vi "Configure Outputs.vi"(0 "VISA resource name":refnum<visa-resource-name>, 1 "Analog Bandwidth (0: bw200kHz)":i32(ring) items=["bw200kHz", "bw50kHz", "bw25kHz"], 2 "Sample Rate (24000 Hz)":dbl=24000.0, 5 "Domain (0: odAnalog)":i32(ring) items=["odAnalog", "odDigital", "odExternal"], 7 "Channels (1)":i32=1, 9 "Connector Type (0: cXLR)":i32(ring) items=["cXLR", "cBNC", "cOptical"], 11 "error in (no error)":errorcluster, 12 "Enable Digital Dual Connector (T: Enable)":bool=TRUE) -> (4 "VISA resource name out":refnum<visa-resource-name>, 15 "error out":errorcluster)   [LabVIEW 2014, in "Stanford Research SR1.lvlib"]
doc: "Configures the attributes for the Quick Measurement Outputs."
uses:
  Stanford Research SR1.lvlib
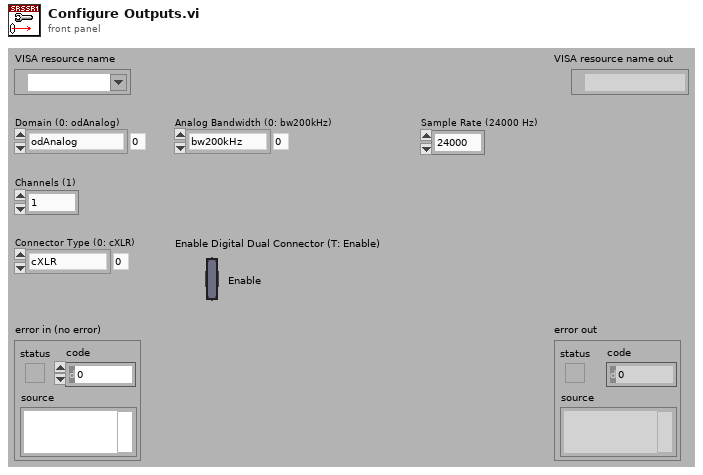
[diagram p1: front panel]
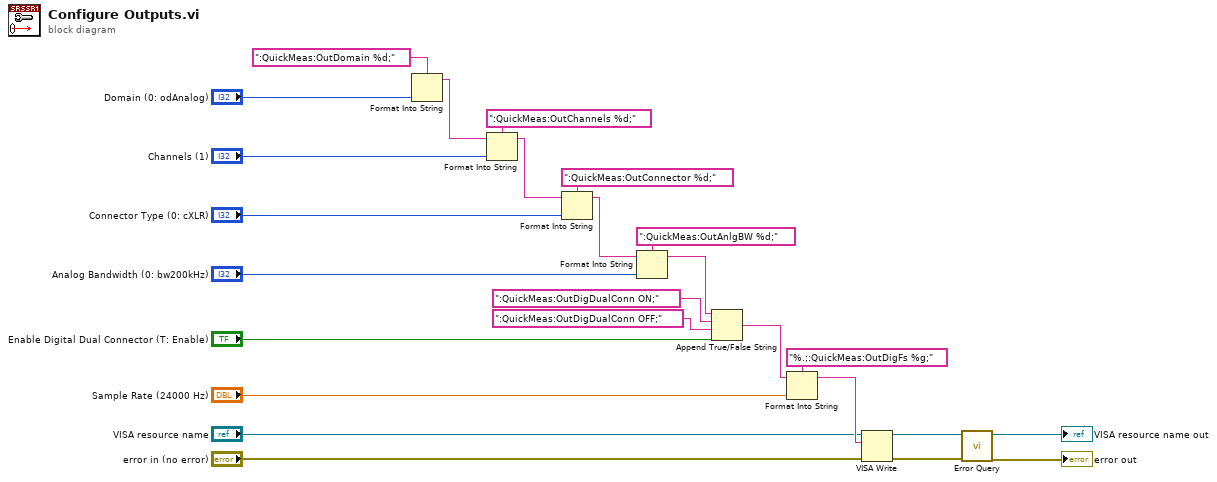
[diagram p0: block diagram]
diagram:
  n1 = Format Into String(format string=":QuickMeas:OutDomain %d;", "Domain (0: odAnalog)") -> (resulting string=w23:string)  [unwired: 2 in, 1 out]
  n2 = Format Into String(format string=":QuickMeas:OutChannels %d;", initial string=w23, "Channels (1)") -> (resulting string=w20:string)  [unwired: 1 in, 1 out]
  n3 = Format Into String(format string=":QuickMeas:OutConnector %d;", initial string=w20, "Connector Type (0: cXLR)") -> (resulting string=w17:string)  [unwired: 1 in, 1 out]
  n4 = Format Into String(format string=":QuickMeas:OutAnlgBW %d;", initial string=w17, "Analog Bandwidth (0: bw200kHz)") -> (resulting string=w14:string)  [unwired: 1 in, 1 out]
  n5 = Append True/False String(1:"Enable Digital Dual Connector (T: Enable)", 2:":QuickMeas:OutDigDualConn OFF;", 3:":QuickMeas:OutDigDualConn ON;", 4:w14) -> (0:w10:string)
  n6 = Format Into String(format string="%.;:QuickMeas:OutDigFs %g;", initial string=w10, "Sample Rate (24000 Hz)") -> (resulting string=w7:string)  [unwired: 1 in, 1 out]
  n7 = VISA Write(VISA resource name="VISA resource name", write buffer=w7, error in (no error)="error in (no error)") -> (VISA resource name out=w4:refnum<visa-resource-name>, error out=w3:errorcluster)  [unwired: 1 out]
  n8 = call "Error Query.vi"("error in (no error)"=w3, "VISA resource name"=w4) -> ("error out"=→"error out":errorcluster, "VISA resource name out"=→"VISA resource name out":refnum<visa-resource-name>)  [unwired: 6 in, 2 out]
